vi "DatabaseHand_Delete.vi"(8 "error in (no error)":errorcluster, 10 "name":string, 11 "Database RefNum in":T1) -> (0 "error out":errorcluster, 1 "type":string, 2 "value":string, 3 "Database RefNum out":T1, 4 "permissions":string="RW", 6 "unit":string)   [LabVIEW 2016]
doc: "This VI finds the RefNum of an existing object with the input Name or creates a new object if the Name is not found or Name is unwired or an empty string.\nCopyright 2001 VI Engineering, Inc."
uses:
  private/vis/DatabaseHand_RefNum.ctl
  private/vis/DatabaseHand_Function.ctl
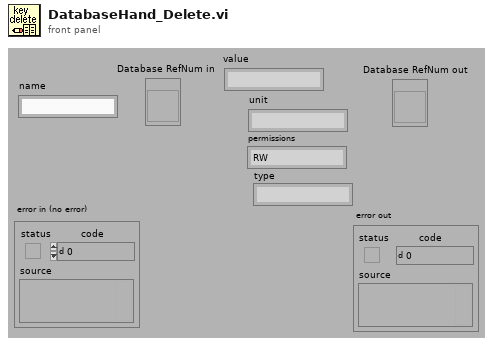
[diagram p1: front panel]
types:
  T1 = typedef "DatabaseHand_RefNum.ctl" = refnum<vi>
  T2 = typedef "DatabaseHand_Function.ctl" = enum16{"Reset", "Register", "Get Data", "Set Data", "Unregister", "Test", "Get Objects", "Delete Data"}
  T3 = typedef "DatabaseHand_Element.ctl" = cluster{"name":string, "Database":T4[]}
  T4 = typedef "DatabaseHan_DatabaseElement.ctl" = cluster{"name":string, "value":string, "type":string, "unit":string, "permissions":string, "enqueued":bool, "group":string}
  T5 = typedef "Database_Refnum.ctl" = refnum<vi>
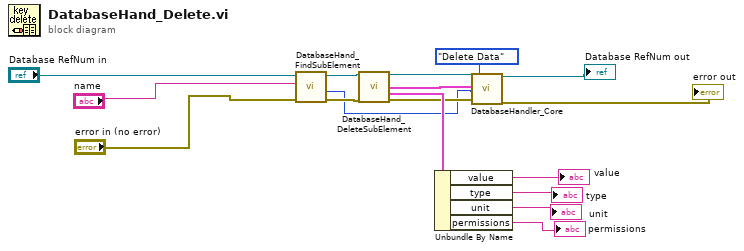
[diagram p0: block diagram]
diagram:
  n1 = call "DatabaseHand_FindSubElement.vi"("error in (no error)"="error in (no error)", "name"="name", "Database RefNum in"="Database RefNum in") -> ("error out"=w14:errorcluster, "index"=w1:i32, "Database RefNum out"=w13:T1)  [unwired: 6 out]
  n2 = call "DatabaseHand_DeleteSubElement.vi"("Database RefNum in"=w13, "error in (no error)"=w14) -> ("Database RefNum out"=w5:T1, "Object Data Out"=w3:T3, "Element deleted"=w8:T4, "error out"=w7:errorcluster)  [unwired: 2 in, 8 out]
  n3 = Unbundle By Name(w8) -> ("value"=→"value":string, "type"=→"type":string, "unit"=→"unit":string, "permissions"=→"permissions":string)
  n4 = call "DatabaseHandler_Core.vi"("Object Refnum In"=w5, "Object Data In"=w3, "subele index"=w1, "error in (no error)"=w7, "Function (Get Data)"=DatabaseHand_Function."Delete Data") -> ("Object Refnum out"=→"Database RefNum out":T5, "error out"=→"error out":errorcluster)  [unwired: 2 in, 11 out]
